vi "OAT Tachless Speed Profile Generator.vi"(8 "error in (no error)":errorcluster, 11 "scaled signal [EU]":waveform(dbl)={"t0"=timestamp(0 s since 1904-01-01), "dt"=0.0, "Y"=[]}) -> (0 "error out":errorcluster, 1 "orders list":dbl[](array[numeric]) format="%.2f", 2 "speed profile":T2 {"speed [RPM]" format="%.2f"; "time [s]" format="%.2f"}, 3 "dup scaled signal [EU]":waveform(dbl), 4 "window info":T3={"window type"=62, "window length"=2048} {"window type" items=["None"=0, "Hanning"=1, "Hamming"=2, "Blackman-Harris"=3, "Exact Blackman"=4, "Blackman"=5, "Flat Top"=6, "4 Term B-Harris"=7, "7 Term B-Harris"=8, "Low Sidelobe"=9, "Gaussian"=62]; "window length" min=0}, 5 "effective bandwidth":T1={"bandwidth value"=0.5, "bandwidth unit"=enum."Order"} {"bandwidth value" min=0.0 format="%.2f"})   [LabVIEW 2017, in "SoundVib_Tachless.lvlib"]
doc: "Generates a speed profile from a sound or vibration signal without a tachometer signal. This VI launches an interactive configuration dialogue that must be configured each time the VI is run."
uses:
  <vilib>/addons/Sound and Vibration/Order Analysis/Tachless/SoundVib_Tachless.lvlib
  <vilib>/addons/Sound and Vibration/Order Analysis/Ref Gabor Order Tracking/window information.ctl
  <vilib>/addons/Sound and Vibration/Order Analysis/Tach Process/SubVIs/speed profile.ctl
  <vilib>/addons/Sound and Vibration/Order Analysis/Ref Gabor Order Tracking/Mask Bandwidth.ctl
  <vilib>/addons/Sound and Vibration/Order Analysis/Gabor Order Tracking/SoundVib_Gabor.lvlib
  <vilib>/addons/Sound and Vibration/Order Analysis/Tach Process/SoundVib_TachProcess.lvlib
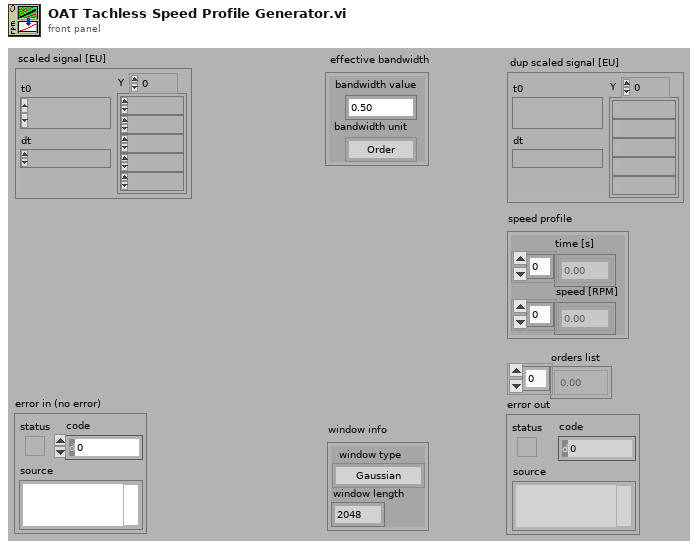
[diagram p1: front panel]
types:
  T1 = typedef "SoundVib_Gabor.lvlib/Mask Bandwidth.ctl" = cluster{"bandwidth value":dbl, "bandwidth unit":enum16{"Order", "Hz"}}
  T2 = typedef "SoundVib_TachProcess.lvlib/speed profile.ctl" = cluster{"time [s]":dbl[], "speed [RPM]":dbl[]}
  T3 = typedef "SoundVib_Gabor.lvlib/window information.ctl" = cluster{"window type":u32, "window length":i32}
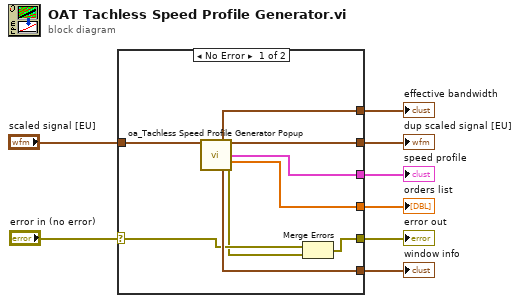
[diagram p0: block diagram]
diagram:
  n1 = case shown="No Error" "error in (no error)" {
    selector: "error in (no error)" -> [w11 w19]
    tunnel: "scaled signal [EU]" -> [w17 w18]
    tunnel: [w9 w19] -> w6
    tunnel: [w16 _] -> w1
    tunnel: [w15 w18] -> w5
    tunnel: [w14 _] -> w4
    tunnel: [w13 _] -> w3
    tunnel: [w12 _] -> w2
    frame No Error {
      n2 = call <vilib>:"oa_Tachless Speed Profile Generator Popup.vi"("scaled signal [EU]"=w17) -> ("effective bandwidth"=w16:T1, "dup scaled signal [EU]"=w15:waveform(dbl), "speed profile"=w14:T2, "orders list"=w13:dbl[], "window info"=w12:T3, "error out"=w10:errorcluster)  [unwired: 9 in]
      n3 = Merge Errors(w11, w10) -> (w9:errorcluster)
    }
    frame Error {
    }
  }
  "window info" <- w2
  "speed profile" <- w4
  "orders list" <- w3
  "effective bandwidth" <- w1
  "error out" <- w6
  "dup scaled signal [EU]" <- w5
